vi "Read Test Param.vi"(8 "error in (no error)":errorcluster, 11 "Test Switch Consumer in":refnum<class "Test Switch Consumer.lvclass">) -> (0 "error out":errorcluster, 2 "Test Param":string, 3 "Test Switch Consumer out":refnum<class "Test Switch Consumer.lvclass">)   [LabVIEW 2017, in "Test Switch Consumer.lvclass"]
uses:
  Test Switch Consumer.lvclass
  Test Switch Consumer.lvclass/Test Switch Consumer.ctl
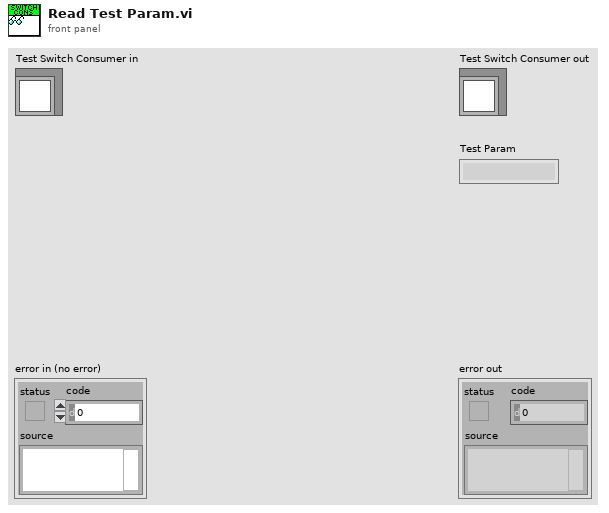
[diagram p1: front panel]
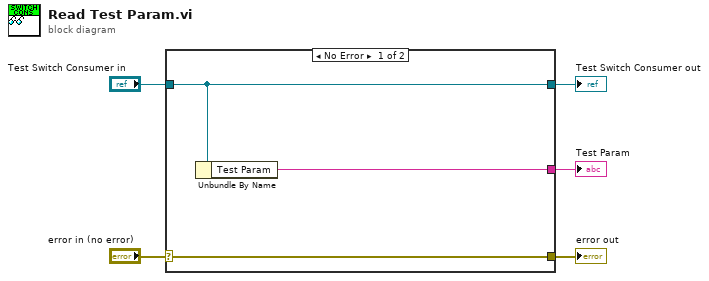
[diagram p0: block diagram]
diagram:
  n1 = case shown="No Error" "error in (no error)" {
    selector: "error in (no error)" -> [w8 w9]
    tunnel: [w8 w9] -> w4
    tunnel: [w7 w10] -> w2
    tunnel: "Test Switch Consumer in" -> [w7 w10]
    tunnel: [w6 _] -> w1
    frame No Error {
      n2 = Unbundle By Name(w7) -> ("Test Param"=w6:string)
    }
    frame Error {
    }
  }
  "error out" <- w4
  "Test Switch Consumer out" <- w2
  "Test Param" <- w1
